vi "ZCAN_TransmitLIN.vi"(0 "lin_index_handle":u32, 5 "error in (no error)":errorcluster caption="错误输入（无错误）", 9 "ZCAN_LIN_MSG":T1) -> (19 "error out":errorcluster caption="错误输出")   [LabVIEW 2020, in "zlgcan.lvlib"]
doc: "该函数用于发送CAN报文。"
uses:
  zlgcan.lvlib
  bin/zlgcan_wrap.dll
  ZCAN_LIN_MSG.ctl
panel:
  in  "每次发送帧数（默认1）":u32=1
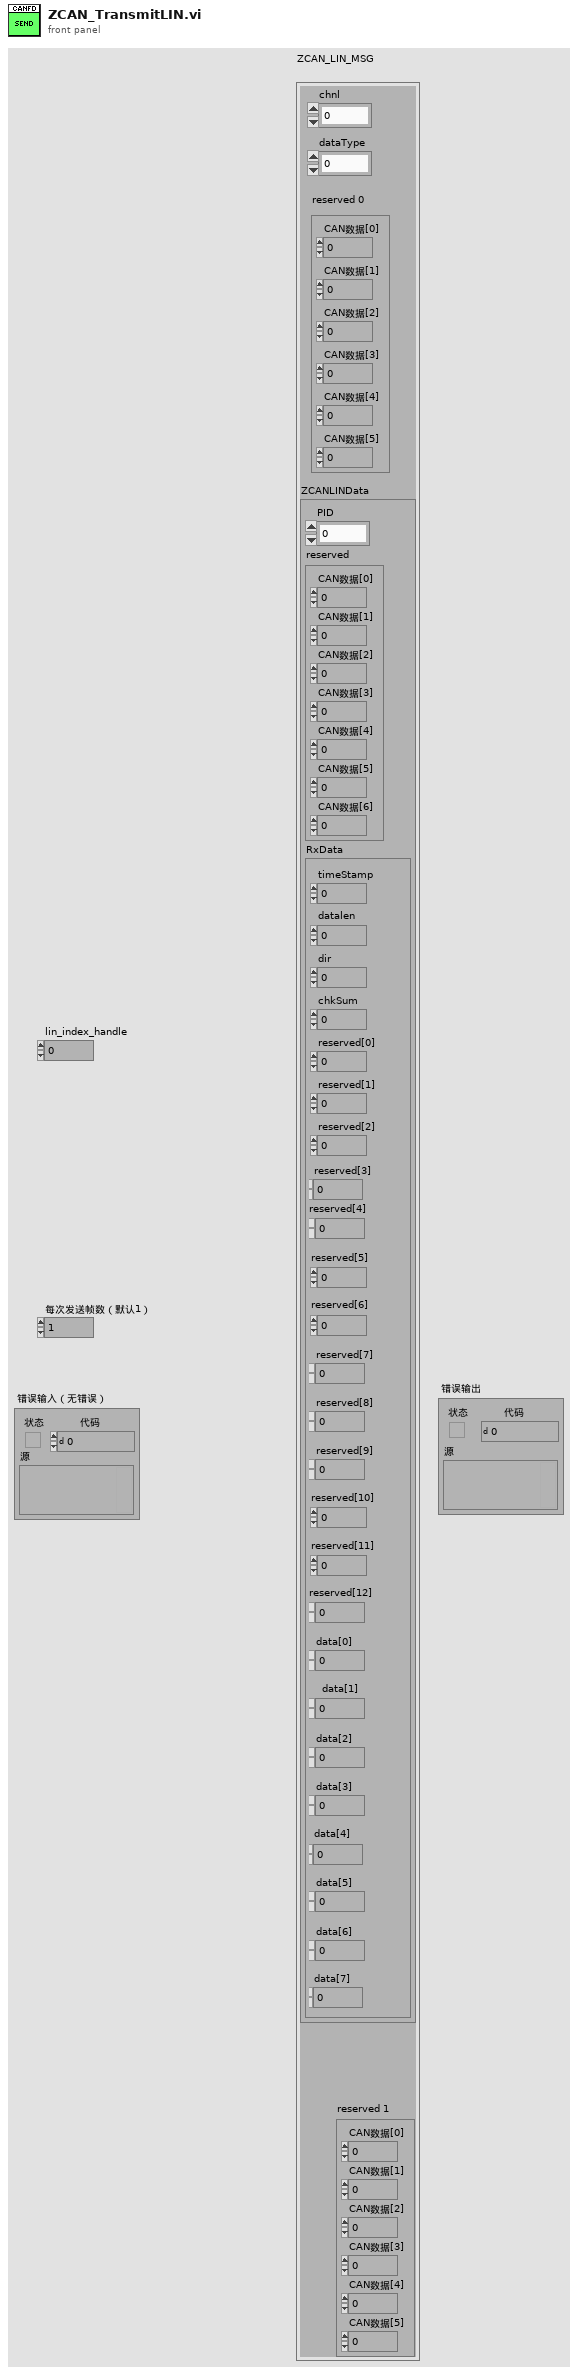
[diagram p1: front panel]
types:
  T1 = typedef "zlgcan.lvlib/ZCAN_LIN_MSG.ctl" = cluster{"chnl":u8, "dataType":u8, "reserved 0":cluster{"CAN数据[0]":u8, "CAN数据[1]":u8, "CAN数据[2]":u8, "CAN数据[3]":u8, "CAN数据[4]":u8, "CAN数据[5]":u8}, "ZCANLINData":cluster{"PID":u8, "reserved":cluster{"CAN数据[0]":u8, "CAN数据[1]":u8, "CAN数据[2]":u8, "CAN数据[3]":u8, "CAN数据[4]":u8, "CAN数据[5]":u8, "CAN数据[6]":u8}, "RxData":cluster{"timeStamp":u64, "datalen":u8, "dir":u8, "chkSum":u8, "reserved[0]":u8, "reserved[1]":u8, "reserved[2] ":u8, "reserved[3]":u8, "reserved[4]":u8, "reserved[5]":u8, "reserved[6] ":u8, "reserved[7] ":u8, "reserved[8]":u8, "reserved[9] ":u8, "reserved[10] ":u8, "reserved[11] ":u8, "reserved[12] ":u8, "data[0]":u8, "data[1]":u8, "data[2]":u8, "data[3]":u8, "data[4]":u8, "data[5]":u8, "data[6]":u8, "data[7]":u8}}, "reserved 1":cluster{"CAN数据[0]":u8, "CAN数据[1]":u8, "CAN数据[2]":u8, "CAN数据[3]":u8, "CAN数据[4]":u8, "CAN数据[5]":u8}}
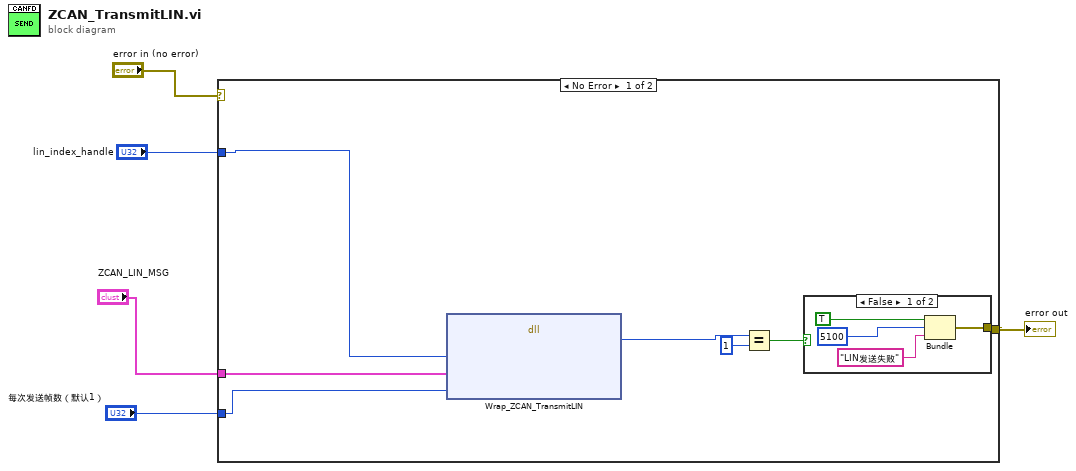
[diagram p0: block diagram]
diagram:
  n1 = case shown="No Error" "error in (no error)" {
    selector: "error in (no error)" -> [_ w17]
    tunnel: [w12 w17] -> w4
    tunnel: "每次发送帧数（默认1）" -> [w8 _]
    tunnel: "lin_index_handle" -> [w11 _]
    tunnel: "ZCAN_LIN_MSG" -> [w7 _]
    frame No Error {
      n2 = dll-call lib="E:/Jabil tools/JabilTestLib/ZLG_CANFD/bin/zlgcan_wrap.dll" fn="Wrap_ZCAN_TransmitLIN"("通道句柄"=w11, "数据帧数组"=w7, "数据帧数"=w8) -> ("返回类型"=w10:u32)  [unwired: 6 in, 2 out]
      n3 = Equal?(x=w10, y=u32 1) -> (x = y?=w9:bool)
      n4 = case shown="False" w9 {
        tunnel: [w13 _] -> w12
        frame False {
          n5 = Bundle("status"=TRUE, "code"=5100, "消息"="LIN发送失败") -> (w13:cluster{"status":bool, "code":i32, "消息":string})  [unwired: 1 in]
        }
        frame True {
        }
      }
    }
    frame Error {
    }
  }
  "error out" <- w4
